vi "Read Serialized.vi"(8 "error in (no error)":errorcluster, 11 "Pulse Train in":refnum<class "Pulse Train.lvclass">) -> (0 "error out":errorcluster, 2 "Serialized":T1, 3 "Pulse Train out":refnum<class "Pulse Train.lvclass">)   [LabVIEW 2020, in "Pulse Train.lvclass"]
uses:
  Pulse Train.lvclass
  Serialized.ctl
  Pulse Train.lvclass/Pulse Train.ctl
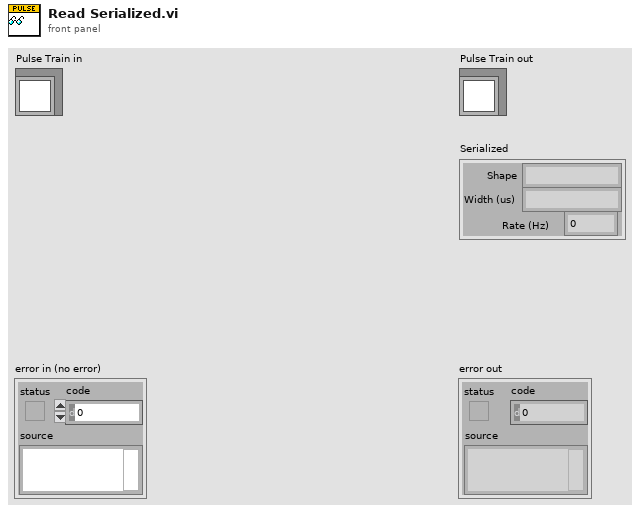
[diagram p1: front panel]
types:
  T1 = typedef "Pulse Train.lvclass/Serialized.ctl" = cluster{"Shape":string, "Width (us)":string, "Rate (Hz)":dbl}
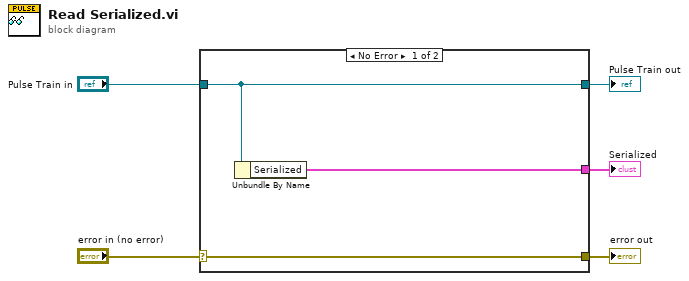
[diagram p0: block diagram]
diagram:
  n1 = case shown="No Error" "error in (no error)" {
    selector: "error in (no error)" -> [w8 w9]
    tunnel: [w8 w9] -> w4
    tunnel: [w7 w10] -> w2
    tunnel: "Pulse Train in" -> [w7 w10]
    tunnel: [w6 _] -> w1
    frame No Error {
      n2 = Unbundle By Name(w7) -> ("Serialized"=w6:T1)
    }
    frame Error {
    }
  }
  "error out" <- w4
  "Pulse Train out" <- w2
  "Serialized" <- w1
